vi "Get USB Strings.vi"(8 "error in (no error)":errorcluster, 11 "RTL-SDR in":refnum<class "RTL-SDR.lvclass">) -> (0 "error out":errorcluster, 1 "function return":i32, 2 "Device USB Strings":T1, 3 "RTL-SDR out":refnum<class "RTL-SDR.lvclass">)   [LabVIEW 2015, in "RTL-SDR.lvclass"]
doc: "Created IvanLis by LabVIEW Portal\nProfile: http://labviewportal.org/memberlist.php?mode=viewprofile&u=987\neMail: IvanLisanov@gMail.com\nTelegram: https://t.me/IvanLis"
uses:
  RTL-SDR.lvclass
  TypeDef/Device USB String.ctl
  RTL-SDR.lvclass/RTL-SDR.ctl
panel:
  in  "manufact":string
  in  "product":string
  in  "serial":string
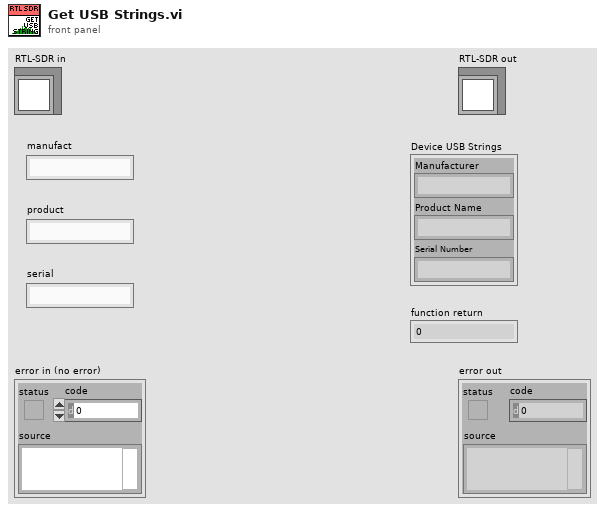
[diagram p1: front panel]
types:
  T1 = typedef "RTL-SDR.lvclass/Device USB String.ctl" = cluster{"Manufacturer":string, "Product Name":string, "Serial Number":string}
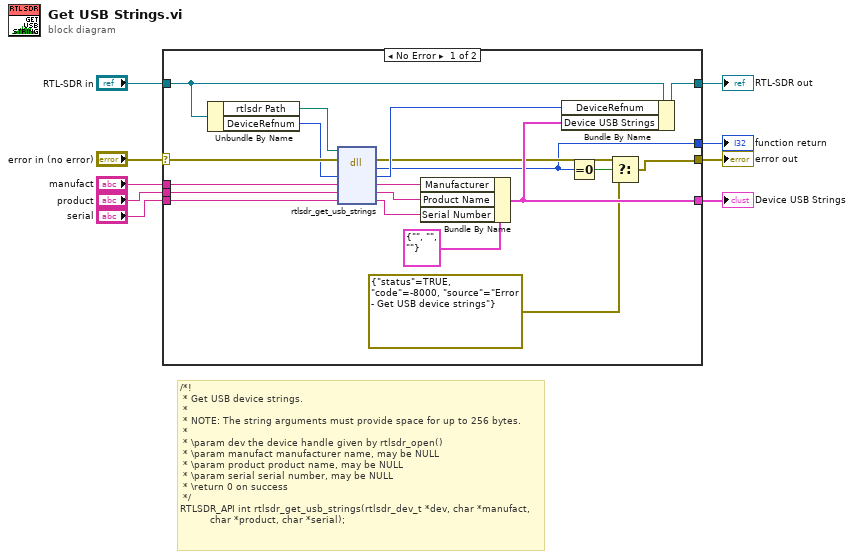
[diagram p0: block diagram]
diagram:
  # "/*!\n * Get USB device strings.\n *\n * NOTE: The string arguments must provide space for up to 256 bytes.\n *\n * \\param dev the device handle given by rtlsdr_open()\n * \\param manufact manufacturer name, may be NULL\n * \\param product product name, may be NULL\n * \\param serial serial number, may be NULL\n * \\return 0 on success\n */\nRTLSDR_API int rtlsdr_get_usb_strings(rtlsdr_dev_t *dev, char *manufact,\n\t\t\t\t      char *product, char *serial);"
  n1 = case shown="No Error" "error in (no error)" {
    selector: "error in (no error)" -> [w28 w30]
    tunnel: [w11 w30] -> w8
    tunnel: [w26 w29] -> w6
    tunnel: "RTL-SDR in" -> [w27 w29]
    tunnel: [w10 _] -> w5
    tunnel: "manufact" -> [w22 _]
    tunnel: "product" -> [w21 _]
    tunnel: "serial" -> [w20 _]
    tunnel: [w15 _] -> w1
    frame No Error {
      n2 = Unbundle By Name(w27) -> ("rtlsdr Path"=w25:path, "DeviceRefnum"=w24:u64)
      n3 = dll-call lib="C:/Users/Ivan/Desktop/D-23-09-24 (RTL-SDR)/Project (Pelleng-SDR)/RTL-SDR Class/dll/rtlsdr.*" fn="rtlsdr_get_usb_strings"(path in=w25, error in=w28, "DeviceRefnum"=w24, "manufact"=w22, "product"=w21, "serial"=w20) -> (error out=w12:errorcluster, "return type"=w10:i32, "DeviceRefnum"=w23:u64, "manufact"=w18:string, "product"=w17:string, "serial"=w16:string)  [unwired: 1 in, 1 out]
      n4 = Bundle By Name(cluster=T1 {"Manufacturer"="", "Product Name"="", "Serial Number"=""} ("Device USB Strings"), "Manufacturer"=w18, "Product Name"=w17, "Serial Number"=w16) -> (w15:T1)
      n5 = Bundle By Name(cluster=w27, "DeviceRefnum"=w23, "Device USB Strings"=w15) -> (w26:refnum<class "RTL-SDR.lvclass">)
      n6 = Equal To 0?(x=w10) -> (x = 0?=w13:bool)
      n7 = Select(t=w12, s=w13, f=errorcluster {"status"=TRUE, "code"=-8000, "source"="Error - Get USB device strings"} ("error out")) -> (s? t:f=w11:errorcluster)
    }
    frame Error {
    }
  }
  "error out" <- w8
  "RTL-SDR out" <- w6
  "Device USB Strings" <- w1
  "function return" <- w5
